vi "detect cube.vi"(5 "Image 3":T2(plugin-control), 6 "c1":i8, 7 "c2":i8) -> (0 "Image 4":T2(plugin-control), 1 "_x":dbl, 2 "_y":dbl, 3 "Circles":cluster{"x":dbl, "y":dbl, "r":dbl}[](array[cluster]), 4 "Circles 2":cluster{"x":dbl, "y":dbl, "r":dbl}[](array[cluster]))   [LabVIEW 2018]
uses:
  vision info 2.vi
panel:
  out "x 2":dbl[](array[numeric])
  out "y 2":dbl[](array[numeric])
  out "y":dbl[](array[numeric])
  out "x":dbl[](array[numeric])
  out "Circles Calibrated (Shape Detection 1)":T1(array[cluster]) {"Position"."Y" format="%.2f"; "Position"."X" format="%.2f"}
  out "d":i32
  out "Circles (Shape Detection 1)":T1(array[cluster]) {"Position"."Y" format="%.2f"; "Position"."X" format="%.2f"}
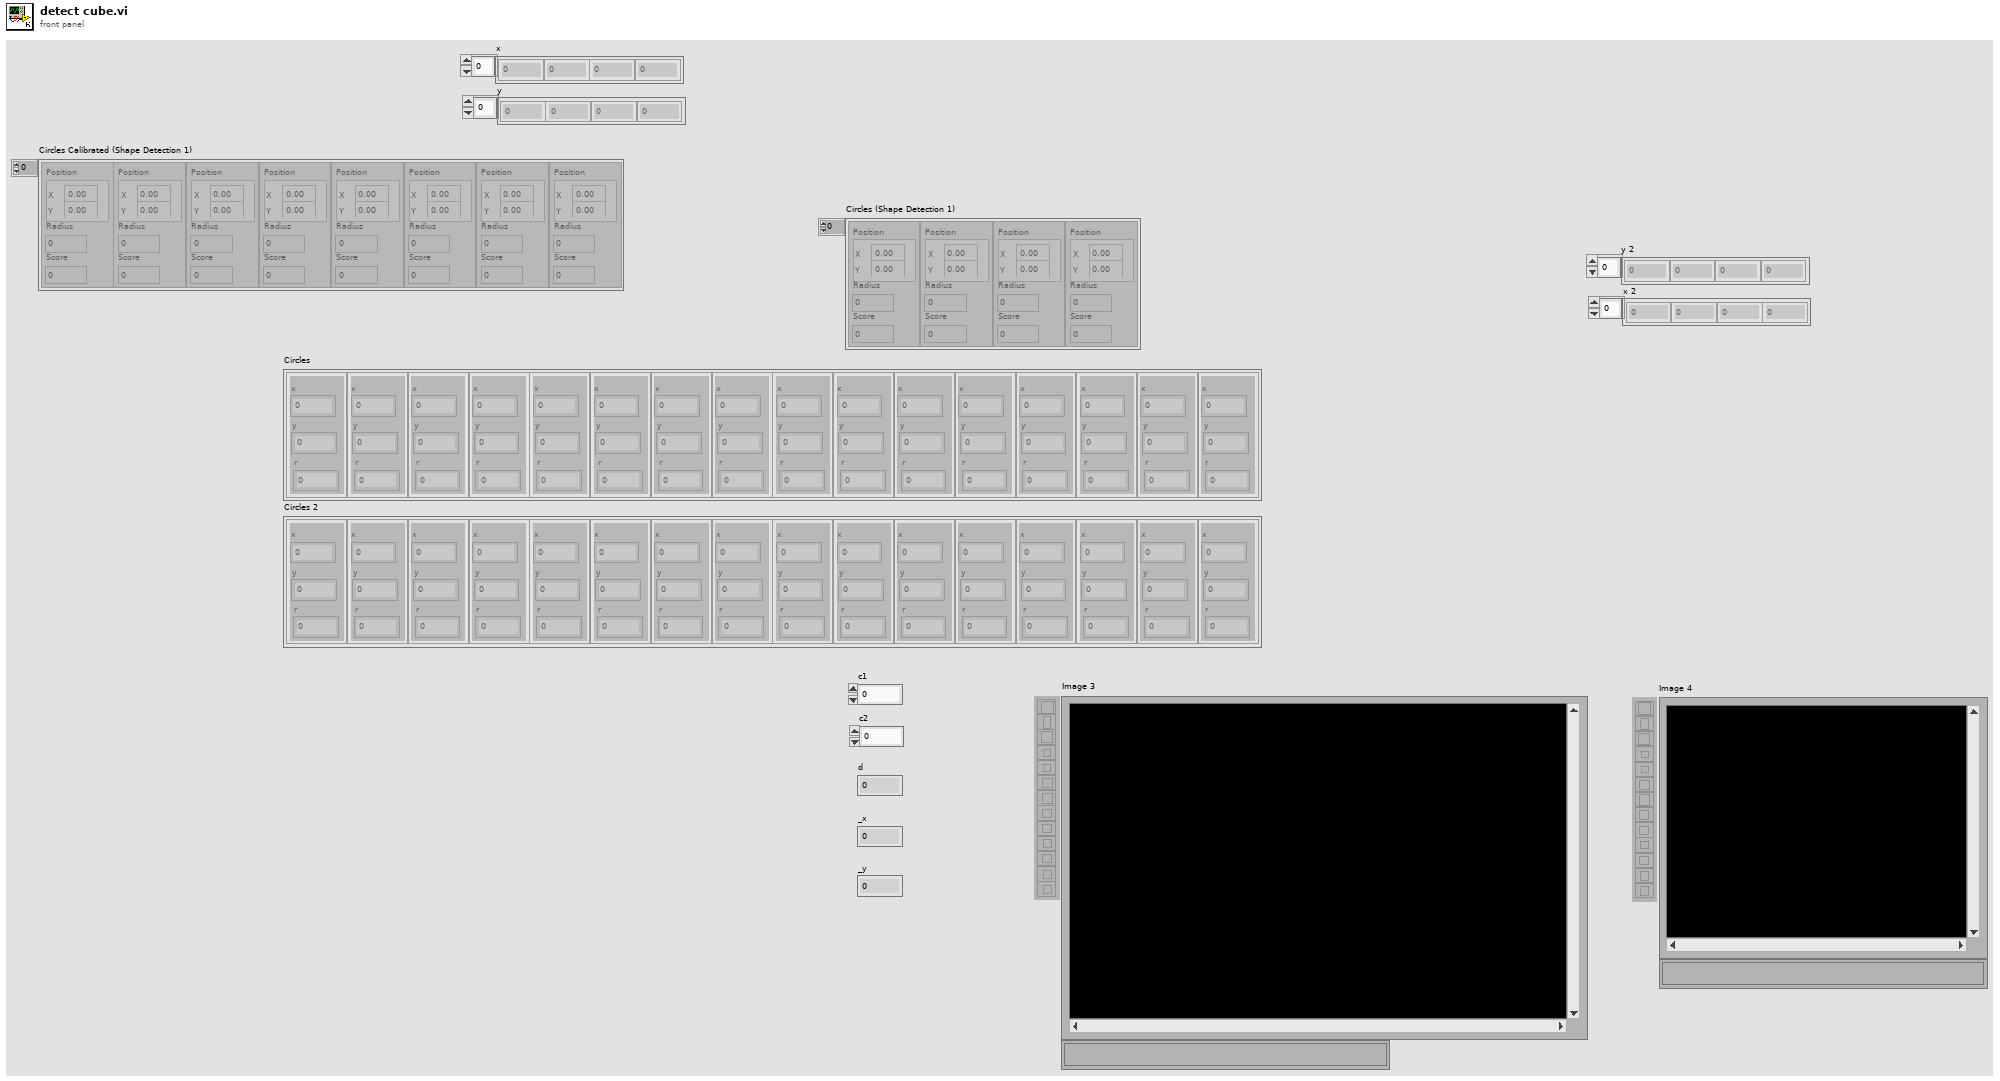
[diagram p1: front panel]
types:
  T1 = cluster{"Position":cluster{"X":sgl, "Y":sgl}, "Radius":dbl, "Score":dbl}[]
  T2 = typedef "IMAQ Image.ctl" = refnum<image>
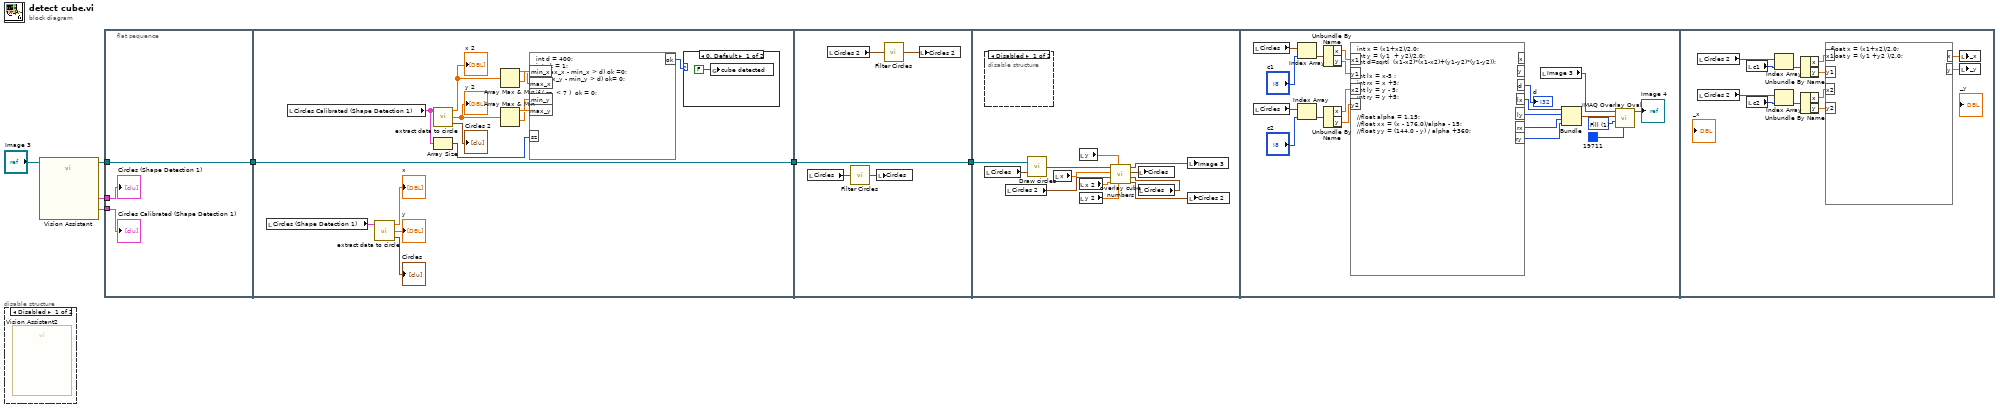
[diagram p0: block diagram]
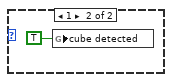
[diagram p3: hidden frame]
diagram:
  n1 = disable-structure shown="Disabled" {
    frame Disabled {
      n2 = call "Vision Assistant2"() -> ()  [unwired: 24 in, 4 out]
    }
    frame Enabled {
    }
  }
  n3 = call "Vision Assistant"("Image In"="Image 3") -> ("Image Out"=w7:T2, "Circles (Shape Detection 1)"=w5:T1, "Circles Calibrated (Shape Detection 1)"=w4:T1)  [unwired: 23 in, 1 out]
  n4 = flat-sequence {
    tunnel: w7 -> [w10]
    tunnel: [w10] -> w3
    tunnel: w5 -> [w9]
    tunnel: w4 -> [w8]
    tunnel: w3 -> [w25]
    tunnel: [w25] -> w2
    tunnel: w2 -> [w32]
    tunnel: [w32] -> w1
    tunnel: w1 -> [w34]
    frame #0 {
      "Circles (Shape Detection 1)" <- w9
      "Circles Calibrated (Shape Detection 1)" <- w8
    }
    frame #1 {
      n5 = local read "Circles (Shape Detection 1)"() -> (w24:T1)
      n6 = local read "Circles Calibrated (Shape Detection 1)"() -> (w12:T1)
      n7 = call "extract data to circle.vi"("Circles (Shape Detection 1)"=w24) -> ("Circles"=→"Circles":cluster{"x":dbl, "y":dbl, "r":dbl}[], "y"=→"y":dbl[], "x"=→"x":dbl[])  [unwired: 2 in]
      n8 = call "extract data to circle.vi"("Circles (Shape Detection 1)"=w12) -> ("Circles"=→"Circles 2":cluster{"x":dbl, "y":dbl, "r":dbl}[], "y"=w19:dbl[], "x"=w18:dbl[])  [unwired: 2 in]
      "y 2" <- w19
      "x 2" <- w18
      n9 = Array Size(array=w12) -> (size(s)=w11:i32)
      n10 = Array Max & Min(array=w18) -> (max value=w14:dbl, min value=w15:dbl)  [unwired: 2 out]
      n11 = Array Max & Min(array=w19) -> (max value=w17:dbl, min value=w16:dbl)  [unwired: 2 out]
      n12 = formula code="int d = 400;\nint ok = 1;\nif (max_x - min_x > d) ok =0;\nif(max_y - min_y > d) ok= 0;\n\nif ( sz  < 7 )  ok = 0;"("min_x"=w15, "max_x"=w14, "min_y"=w16, "max_y"=w17, "sz"=w11) -> ("ok"=w13:i32)
      n13 = case shown="0, Default" w13 {
        frame 0, Default {
          n14 = global write "vision info 2.vi" "cube detected"(FALSE ("cube detected")) -> ()
        }
        frame 1 {
          n15 = global write "vision info 2.vi" "cube detected"(TRUE ("cube detected")) -> ()
        }
      }
    }
    frame #2 {
      n16 = local read "Circles"() -> (w30:cluster{"x":dbl, "y":dbl, "r":dbl}[])
      n17 = local read "Circles 2"() -> (w28:cluster{"x":dbl, "y":dbl, "r":dbl}[])
      n18 = call "Filter Circles.vi"("Circles"=w30) -> ("out"=w31:cluster{"x":dbl, "y":dbl, "r":dbl}[])
      n19 = local write "Circles"(w31) -> ()
      n20 = call "Filter Circles.vi"("Circles"=w28) -> ("out"=w29:cluster{"x":dbl, "y":dbl, "r":dbl}[])
      n21 = local write "Circles 2"(w29) -> ()
    }
    frame #3 {
      n22 = disable-structure shown="Disabled" {
        frame Disabled {
        }
        frame Enabled {
        }
      }
      n23 = local read "Circles"() -> (w35:cluster{"x":dbl, "y":dbl, "r":dbl}[])
      n24 = local read "Circles 2"() -> (w41:cluster{"x":dbl, "y":dbl, "r":dbl}[])
      n25 = call "Draw circles .vi"("Circles"=w35, "Refnum in"=w34) -> ("Refnum out"=w33:T2)
      n26 = local read "x"() -> (w39:dbl[])
      n27 = local read "y"() -> (w38:dbl[])
      n28 = local read "x 2"() -> (w36:dbl[])
      n29 = local read "y 2"() -> (w37:dbl[])
      n30 = local read "Circles"() -> (w43:cluster{"x":dbl, "y":dbl, "r":dbl}[])
      n31 = call "overlay cube numbers.vi"("Circles"=w43, "y 2"=w37, "y"=w38, "x 2"=w36, "Circles 3"=w41, "x"=w39, "Image 2"=w33) -> ("Circles 4"=w40:cluster{"x":dbl, "y":dbl, "r":dbl}[], "Circles 2"=w42:cluster{"x":dbl, "y":dbl, "r":dbl}[], "Image"=w44:T2)
      n32 = local write "Circles"(w42) -> ()
      n33 = local write "Image 3"(w44) -> ()
      n34 = local write "Circles 2"(w40) -> ()
    }
    frame #4 {
      w62 = u32 1 items=["Frame", "Fill"] ("Drawing Mode (Frame)")
      n35 = local read "Circles"() -> (w51:cluster{"x":dbl, "y":dbl, "r":dbl}[])
      n36 = local read "Circles"() -> (w52:cluster{"x":dbl, "y":dbl, "r":dbl}[])
      n37 = Index Array(array=w51, index="c1") -> (element=w50:cluster{"x":dbl, "y":dbl, "r":dbl})
      n38 = Index Array(array=w52, index="c2") -> (element=w49:cluster{"x":dbl, "y":dbl, "r":dbl})
      n39 = Unbundle By Name(w50) -> ("x"=w48:dbl, "y"=w47:dbl)
      n40 = Unbundle By Name(w49) -> ("x"=w46:dbl, "y"=w45:dbl)
      n41 = formula code="int x = (x1+x2)/2.0;\nint y = (y1  + y2)/2.0;\nint d=sqrt(  (x1-x2)*(x1-x2)+(y1-y2)*(y1-y2));\n\nint lx = x-5 ;\nint rx = x +5;\nint ly = y - 5;\nint ry = y +5;\n\n\n//float alpha = 1.15;\n//float xx = (x - 176.0)/alpha - 15;\n//float yy = (144.0 - y) / alpha +360;"("x1"=w48, "y1"=w47, "x2"=w46, "y2"=w45) -> ("d"=→"d":i32, "lx"=w59:i32, "ly"=w58:i32, "rx"=w57:i32, "ry"=w56:i32)  [unwired: 2 out]
      n42 = local read "Image 3"() -> (w53:T2)
      n43 = Bundle(w59, w58, w57, w56) -> (w55:cluster{i32, i32, i32, i32})  [unwired: 1 in]
      n44 = call "IMAQ Overlay Oval"("Color"=u32 19711, "Drawing Mode (Frame)"=w62, "Bounding Rectangle"=w55, "Image"=w53) -> ("Image Out"=→"Image 4":T2)  [unwired: 6 in, 1 out]
    }
    frame #5 {
      n45 = local read "Circles 2"() -> (w75:cluster{"x":dbl, "y":dbl, "r":dbl}[])
      n46 = local read "Circles 2"() -> (w73:cluster{"x":dbl, "y":dbl, "r":dbl}[])
      n47 = local read "c1"() -> (w76:i8)
      n48 = local read "c2"() -> (w74:i8)
      n49 = Index Array(array=w75, index=w76) -> (element=w72:cluster{"x":dbl, "y":dbl, "r":dbl})
      n50 = Index Array(array=w73, index=w74) -> (element=w71:cluster{"x":dbl, "y":dbl, "r":dbl})
      n51 = Unbundle By Name(w72) -> ("x"=w70:dbl, "y"=w69:dbl)
      n52 = Unbundle By Name(w71) -> ("x"=w68:dbl, "y"=w67:dbl)
      n53 = formula code="float x = (x1+x2)/2.0;\nfloat y = (y1 +y2 )/2.0;"("x1"=w70, "y1"=w69, "x2"=w68, "y2"=w67) -> ("x"=w66:dbl, "y"=w65:dbl)
      n54 = local write "_x"(w66) -> ()
      n55 = local write "_y"(w65) -> ()
    }
  }
